vi "service new.vi"() -> ()   [LabVIEW 2009]
uses:
  <vilib>/printing/ReportDocExtensions.llb/Append Front Panel Image to Report (path).vi
  <vilib>/Utility/NIReport.llb/NI_report.lvclass
  <vilib>/Utility/NIReport.llb/NI_ReportGenerationCore.lvlib
panel:
  out "ALL":dbl[](graph)
  out "Left 2":dbl[](graph)
  out "Right":dbl[](graph)
  out "Serve 4":dbl[](graph)
  out "Serve 5":dbl[](graph)
  out "Serve 1":dbl[](graph)
  out "Serve 6":dbl[](graph)
  out "Serve 7":dbl[](graph)
  out "Serve 2":dbl[](graph)
  out "Serve 8":dbl[](graph)
  out "Serve 9":dbl[](graph)
  out "Serve 3":dbl[](graph)
  in  "S1":bool
  in  "TL":bool
  in  "BR":bool
  in  "BL":bool
  in  "BM":bool
  in  "CR":bool
  in  "CM":bool
  in  "CL":bool
  in  "TR":bool
  in  "TM":bool
  in  "1":bool
  in  "2":bool
  in  "3":bool
  in  "S 2":bool
  in  "Code":bool
  in  "stop":bool
  in  "save file to":path=path "C:/Users/Sports Tech/Desktop/kokum/Service VI/SAVED FILES/results.doc"
  in  "String":string
  in  "reset":bool
  in  "Boolean":bool
  in  "SHOW 2 to 2":bool
  in  "SHOW 2 to 1":bool
  in  "SHOW 1 to 2":bool
  in  "SHOW 1 to 1":bool
  in  "Serving 2 to 2":bool
  in  "Serving 2 to 1":bool
  in  "Serving 1 to 2":bool
  in  "Serving 1 to 1":bool
  out "service from right2 to 2":dbl[][](array[numeric])
  out "service from right2 to 1":dbl[][](array[numeric])
  out "service from right1 to 2":dbl[][](array[numeric])
  out "serving from left2 to 2":dbl[][](array[numeric])
  out "serving from left2 to 1":dbl[][](array[numeric])
  out "serving from left1 to 2":dbl[][](array[numeric])
  in  "TEAM 2 Player 2":string
  in  "TEAM 2 Player 1":string
  in  "TEAM 1 Player 2":string
  in  "TEAM 1 Player 1":string
  out "serve3":dbl[][](array[numeric])
  out "serve2":dbl[][](array[numeric])
  out "serve1":dbl[][](array[numeric])
  out "serv1 from right":dbl[][](array[numeric])
  out "serv2 from right":dbl[][](array[numeric])
  out "serv3 from right":dbl[][](array[numeric])
  out "serv3 from left":dbl[][](array[numeric])
  out "serv2 from left":dbl[][](array[numeric])
  out "serv1 from left":dbl[][](array[numeric])
  out "all serves":dbl[][](array[numeric])
  out "service from right1 to 1":dbl[][](array[numeric])
  out "serving from left1 to 1":dbl[][](array[numeric])
  # "SWITCH"
  # "Player position"
  # "Serving"
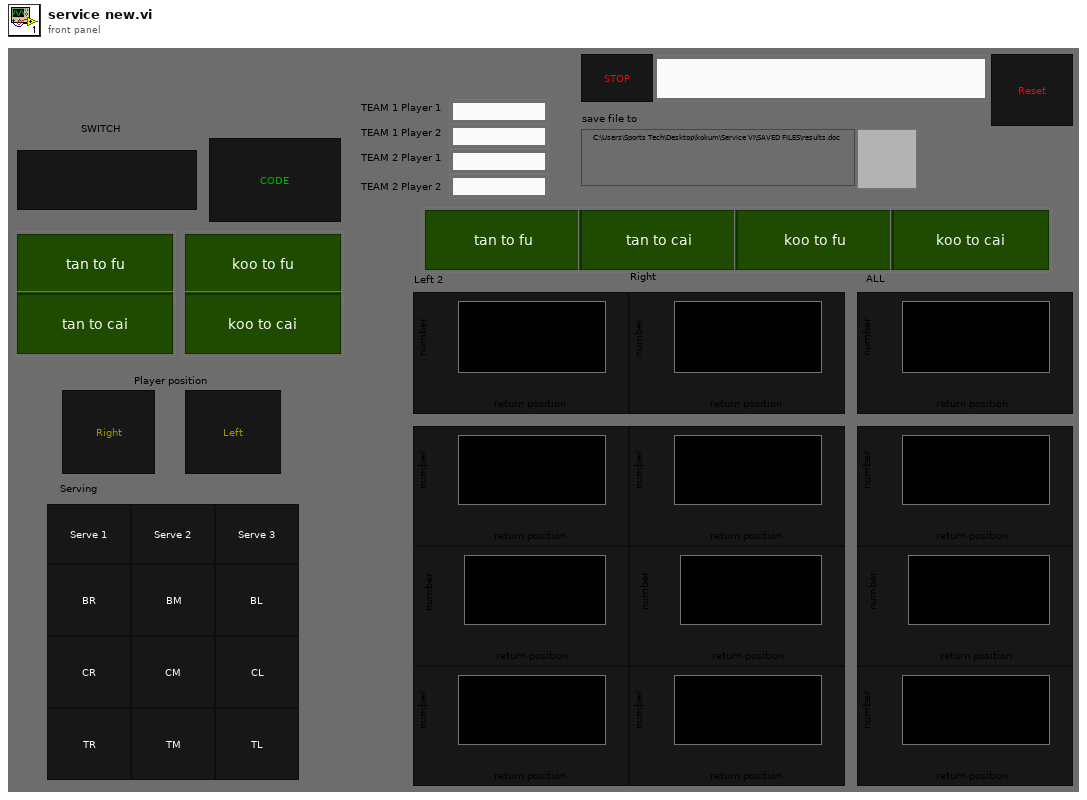
[diagram p1: front panel]
types:
  T1 = typedef "LVPositionTypeDef.ctl" = cluster{"Left":i32, "Top":i32}
  T2 = cluster{"Position":T1, "Position":T1, "Position":T1, "Position":T1, "Position":T1, "Position":T1, "Position":T1, "Position":T1, "Position":T1}
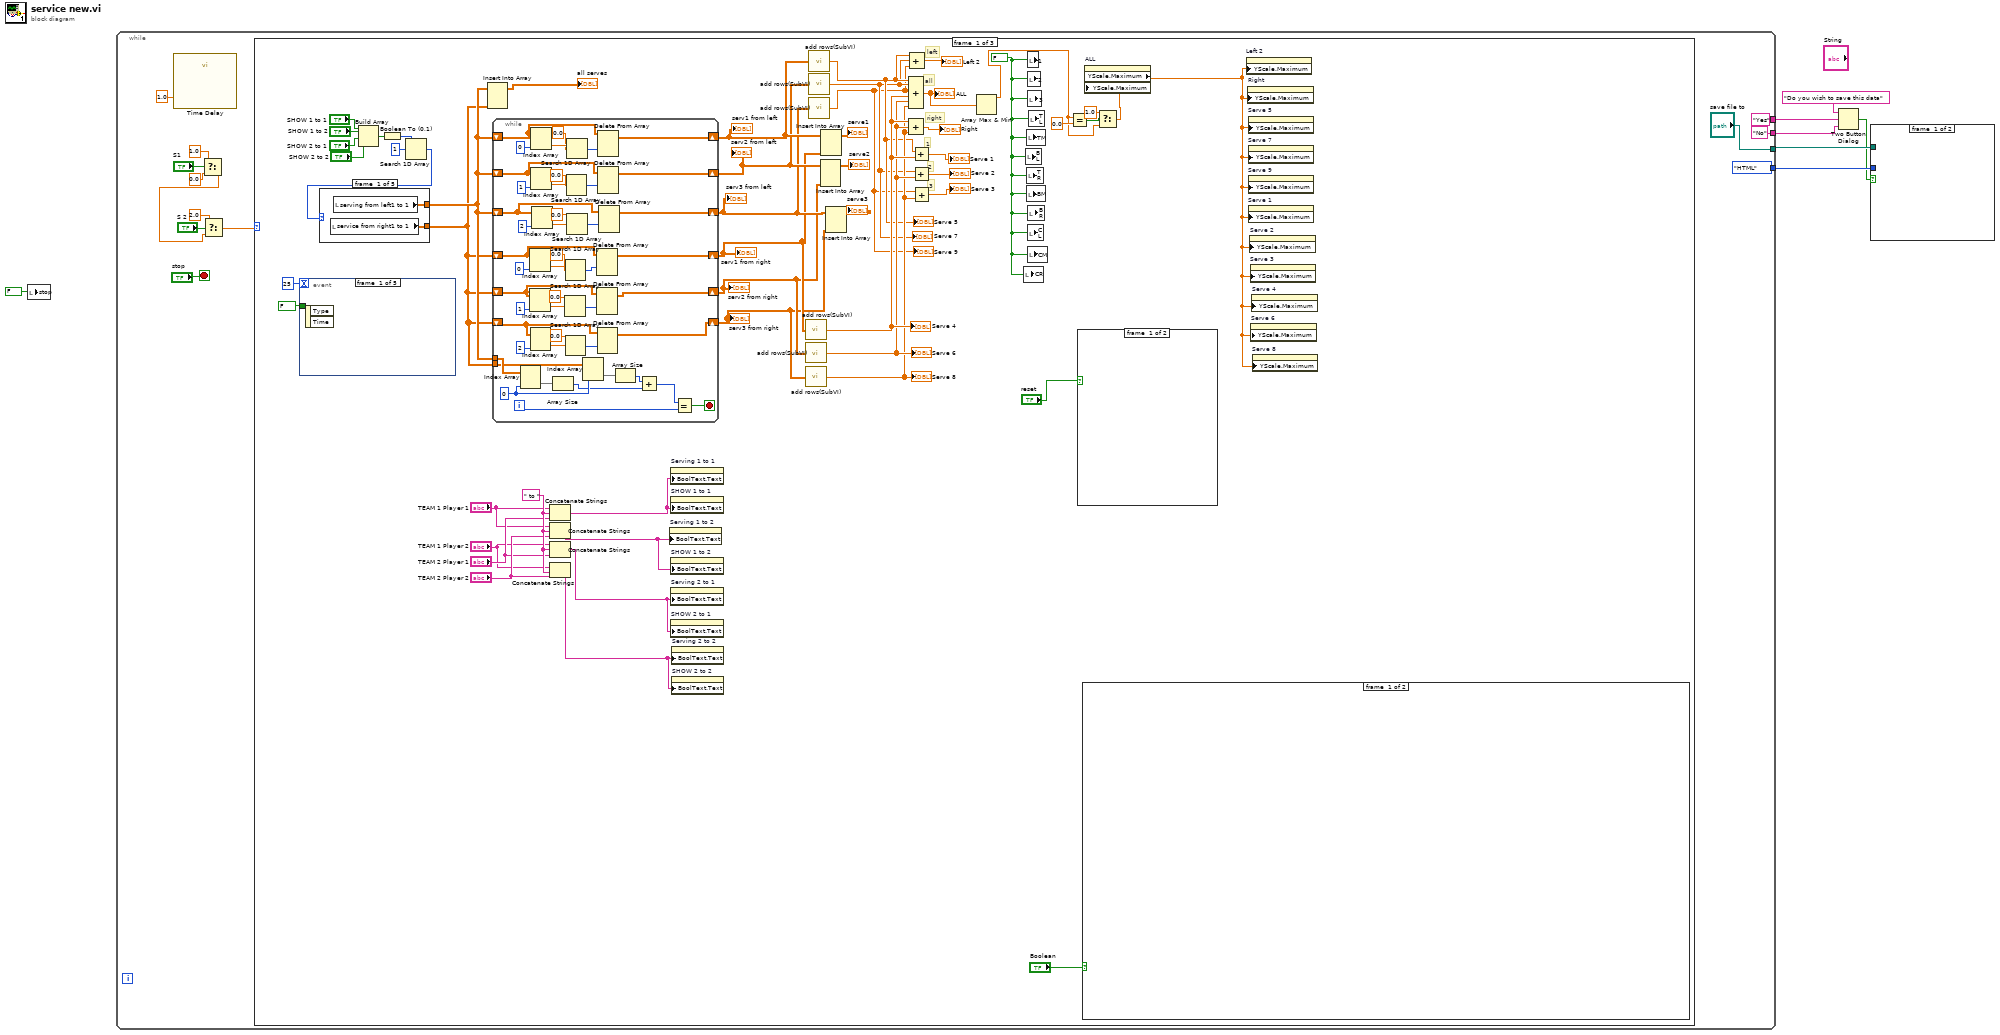
[diagram p0: block diagram]
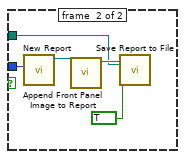
[diagram p2: hidden frame]
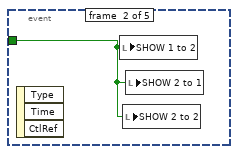
[diagram p3: hidden frame]
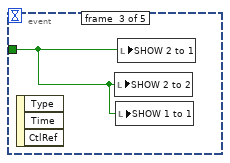
[diagram p4: hidden frame]
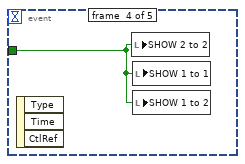
[diagram p5: hidden frame]
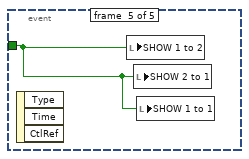
[diagram p6: hidden frame]
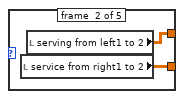
[diagram p7: hidden frame]
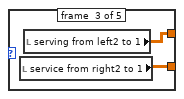
[diagram p8: hidden frame]
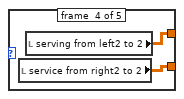
[diagram p9: hidden frame]
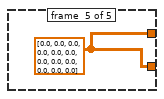
[diagram p10: hidden frame]
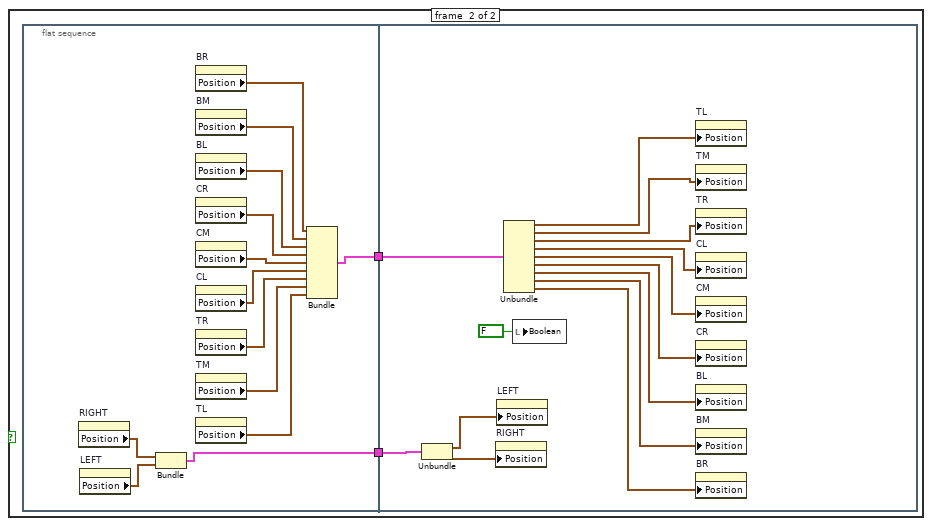
[diagram p11: hidden frame]
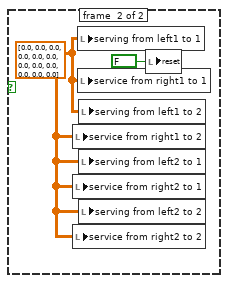
[diagram p12: hidden frame]
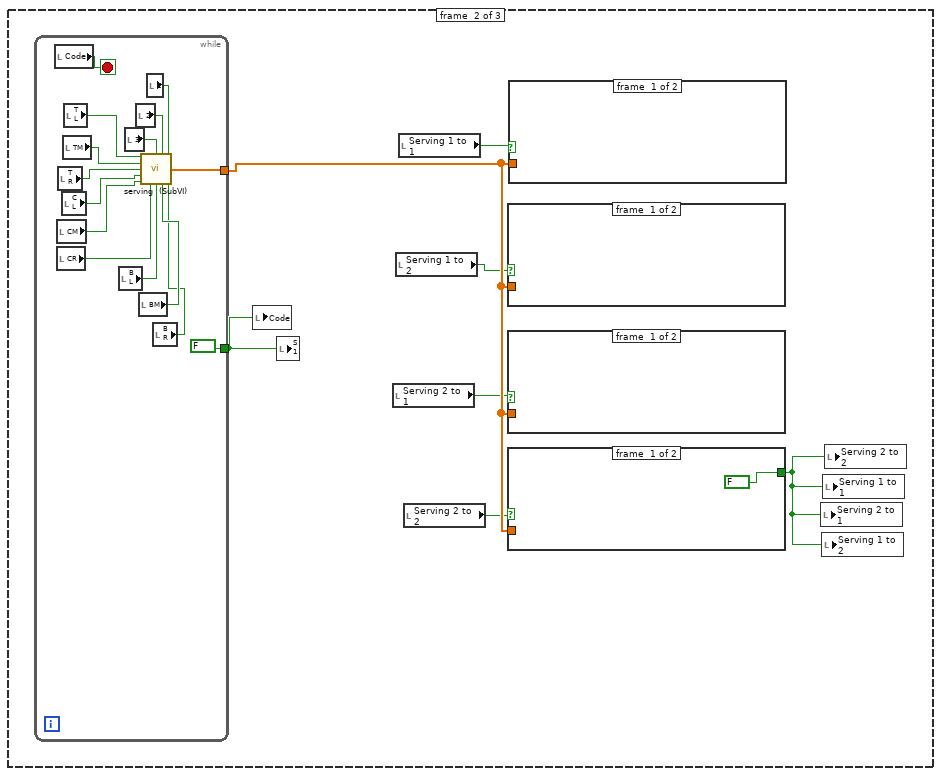
[diagram p13: hidden frame]
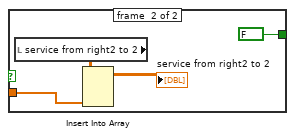
[diagram p14: hidden frame]
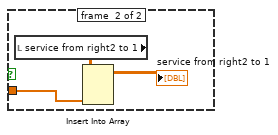
[diagram p15: hidden frame]
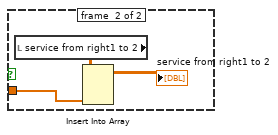
[diagram p16: hidden frame]
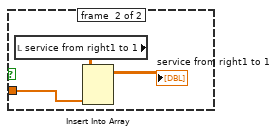
[diagram p17: hidden frame]
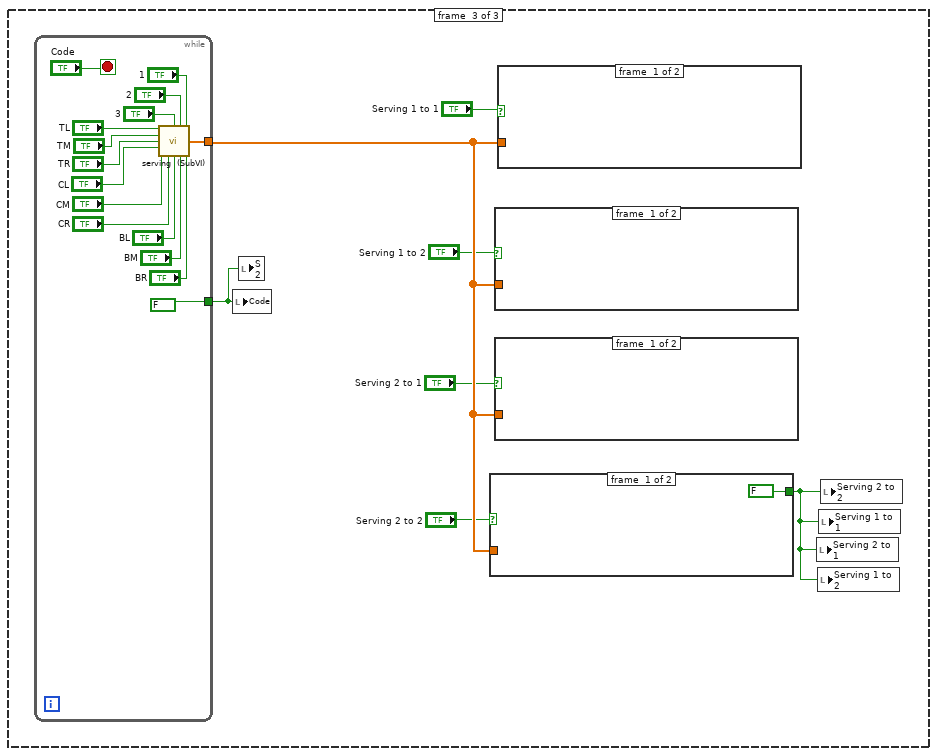
[diagram p18: hidden frame]
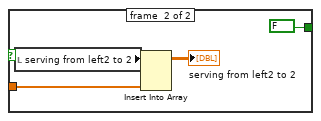
[diagram p19: hidden frame]
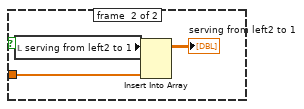
[diagram p20: hidden frame]
diagram:
  n1 = local write "stop"(FALSE ("stop")) -> ()
  n2 = while {
    tunnel: [enum16{"Standard Report", "HTML"}."HTML" ("report type")] -> w7
    tunnel: ["save file to"] -> w6
    tunnel: ["Yes" ("T button name (\"OK\")")] -> w3
    tunnel: ["No" ("F button name (\"Cancel\")")] -> w2
    stop <- "stop" stop-if-true
    n3 = call "Time Delay"("Delay Time (s)"=1.0) -> ()  [unwired: 10 in, 1 out]
    n4 = Select(t=1.0, s="S1", f=0.0) -> (s? t:f=w15:dbl)
    n5 = Select(t=2.0, s="S 2", f=w15) -> (s? t:f=w13:dbl)
    n6 = case shown="0, Default" w13 {
      frame #0 {
        w37 = " to " ("string")
        w51 = FALSE ("1")
        # "3"
        # "2"
        # "1"
        # "all"
        # "right"
        # "left"
        n7 = event shown="[4] \"SHOW 2 to 2\": Value Change" {
          selector: _ -> [_ _ _ _ _]
          dyn-events: _ -> [_ _ _ _ _]
          timeout: 25 -> [_ _ _ _ _]
          tunnel: FALSE ("SHOW 1 to 2") -> [_ w73 w74 w75 w76]
          event #0 {
            n8 = event-data() -> ()  [unwired: 1 in, 2 out]
          }
          event #1 {
            n9 = event-data() -> ()  [unwired: 1 in, 3 out]
            n10 = local write "SHOW 1 to 2"(w73) -> ()
            n11 = local write "SHOW 2 to 2"(w73) -> ()
            n12 = local write "SHOW 2 to 1"(w73) -> ()
          }
          event #2 {
            n13 = event-data() -> ()  [unwired: 1 in, 3 out]
            n14 = local write "SHOW 2 to 2"(w74) -> ()
            n15 = local write "SHOW 1 to 1"(w74) -> ()
            n16 = local write "SHOW 2 to 1"(w74) -> ()
          }
          event #3 {
            n17 = event-data() -> ()  [unwired: 1 in, 3 out]
            n18 = local write "SHOW 2 to 2"(w75) -> ()
            n19 = local write "SHOW 1 to 1"(w75) -> ()
            n20 = local write "SHOW 1 to 2"(w75) -> ()
          }
          event #4 {
            n21 = event-data() -> ()  [unwired: 1 in, 3 out]
            n22 = local write "SHOW 1 to 2"(w76) -> ()
            n23 = local write "SHOW 2 to 1"(w76) -> ()
            n24 = local write "SHOW 1 to 1"(w76) -> ()
          }
        }
        n25 = Build Array("SHOW 1 to 1", "SHOW 1 to 2", "SHOW 2 to 1", "SHOW 2 to 2") -> (w28:bool[])
        n26 = Boolean To (0,1)(Boolean=w28) -> (0, 1=w27:i16[])
        n27 = Search 1D Array(1D array=w27, element=i16 1) -> (index of element=w25:i32)  [unwired: 1 in]
        n28 = case shown="3" w25 {
          tunnel: [w78 w80 w82 w84 w85] -> w24
          tunnel: [w77 w79 w81 w83 w85] -> w23
          frame #0 {
            n29 = local read "service from right1 to 1"() -> (w77:dbl[][])
            n30 = local read "serving from left1 to 1"() -> (w78:dbl[][])
          }
          frame #1 {
            n31 = local read "service from right1 to 2"() -> (w79:dbl[][])
            n32 = local read "serving from left1 to 2"() -> (w80:dbl[][])
          }
          frame #2 {
            n33 = local read "service from right2 to 1"() -> (w81:dbl[][])
            n34 = local read "serving from left2 to 1"() -> (w82:dbl[][])
          }
          frame #3 {
            n35 = local read "service from right2 to 2"() -> (w83:dbl[][])
            n36 = local read "serving from left2 to 2"() -> (w84:dbl[][])
          }
          frame #4 {
            w85 = dbl[][] [[0.0, 0.0, 0.0, 0.0, 0.0, 0.0, 0.0, 0.0, 0.0, 0.0, 0.0, 0.0]] ("serving from left")
          }
        }
        n37 = Insert Into Array(array=w24, new element=w23) -> (→"all serves":dbl[][])  [unwired: 2 in]
        n38 = while {
          shift-right: [w158] -> w68
          shift-left: w24 -> [w160]
          shift-right: [w151] -> w67
          shift-left: w24 -> [w152]
          shift-right: [w146] -> w66
          shift-left: w24 -> [w147]
          shift-right: [w126] -> w65
          shift-left: w23 -> [w129]
          shift-right: [w125] -> w64
          shift-left: w23 -> [w128]
          shift-right: [w124] -> w63
          shift-left: w23 -> [w127]
          tunnel: w24 -> [w123]
          tunnel: w23 -> [w121]
          i -> [w144]
          stop <- w143 stop-if-true
          w122 = 0 ("disabled index (col)")
          n39 = Index Array(array=w123, index (col)=w122) -> (element=w120:dbl[])  [unwired: 1 in]
          n40 = Index Array(array=w129, index (col)=0 ("disabled index (col)")) -> (element=w130:dbl[])  [unwired: 1 in]
          n41 = Index Array(array=w128, index (col)=1 ("disabled index (col)")) -> (element=w135:dbl[])  [unwired: 1 in]
          n42 = Index Array(array=w127, index (col)=2 ("disabled index (col)")) -> (element=w141:dbl[])  [unwired: 1 in]
          n43 = Index Array(array=w160, index (col)=0 ("disabled index (col)")) -> (element=w162:dbl[])  [unwired: 1 in]
          n44 = Index Array(array=w152, index (col)=1 ("disabled index (col)")) -> (element=w155:dbl[])  [unwired: 1 in]
          n45 = Index Array(array=w147, index (col)=2 ("disabled index (col)")) -> (element=w145:dbl[])  [unwired: 1 in]
          n46 = Array Size(array=w120) -> (size(s)=w118:i32)
          n47 = Search 1D Array(1D array=w135, element=0.0) -> (index of element=w133:i32)  [unwired: 1 in]
          n48 = Search 1D Array(1D array=w130, element=0.0) -> (index of element=w132:i32)  [unwired: 1 in]
          n49 = Search 1D Array(1D array=w141, element=0.0) -> (index of element=w139:i32)  [unwired: 1 in]
          n50 = Search 1D Array(1D array=w155, element=0.0) -> (index of element=w157:i32)  [unwired: 1 in]
          n51 = Search 1D Array(1D array=w162, element=0.0) -> (index of element=w159:i32)  [unwired: 1 in]
          n52 = Search 1D Array(1D array=w145, element=0.0) -> (index of element=w149:i32)  [unwired: 1 in]
          n53 = Index Array(array=w121, index (col)=w122) -> (element=w142:dbl[])  [unwired: 1 in]
          n54 = Delete From Array(array=w129, index (row)=w132) -> (array with subset deleted=w126:dbl[][])  [unwired: 2 in, 1 out]
          n55 = Delete From Array(array=w128, index (row)=w133) -> (array with subset deleted=w125:dbl[][])  [unwired: 2 in, 1 out]
          n56 = Delete From Array(array=w127, index (row)=w139) -> (array with subset deleted=w124:dbl[][])  [unwired: 2 in, 1 out]
          n57 = Delete From Array(array=w160, index (row)=w159) -> (array with subset deleted=w158:dbl[][])  [unwired: 2 in, 1 out]
          n58 = Delete From Array(array=w152, index (row)=w157) -> (array with subset deleted=w151:dbl[][])  [unwired: 2 in, 1 out]
          n59 = Delete From Array(array=w147, index (row)=w149) -> (array with subset deleted=w146:dbl[][])  [unwired: 2 in, 1 out]
          n60 = Array Size(array=w142) -> (size(s)=w119:i32)
          n61 = Add(x=w119, y=w118) -> (x+y=w117:i32)
          n62 = Equal?(x=w117, y=w144) -> (x = y?=w143:bool)
        }
        "serv1 from left" <- w68
        "serv2 from left" <- w67
        "serv3 from left" <- w66
        "serv1 from right" <- w65
        "serv2 from right" <- w64
        "serv3 from right" <- w63
        n63 = Concatenate Strings("TEAM 1 Player 1", w37, "TEAM 2 Player 1") -> (w38:string)
        n64 = Concatenate Strings("TEAM 1 Player 1", w37, "TEAM 2 Player 2") -> (w39:string)
        n65 = Concatenate Strings("TEAM 1 Player 2", w37, "TEAM 2 Player 1") -> (w40:string)
        n66 = Concatenate Strings("TEAM 1 Player 2", w37, "TEAM 2 Player 2") -> (w41:string)
        n67 = property on="Serving 1 to 2" class="Bool (strict)"("BoolText.Text"=w39) -> ()  [unwired: 2 in, 2 out]
        n68 = property on="Serving 1 to 1" class="Bool (strict)"("BoolText.Text"=w38) -> ()  [unwired: 2 in, 2 out]
        n69 = property on="SHOW 1 to 1" class="Bool (strict)"("BoolText.Text"=w38) -> ()  [unwired: 2 in, 2 out]
        n70 = property on="SHOW 1 to 2" class="Bool (strict)"("BoolText.Text"=w39) -> ()  [unwired: 2 in, 2 out]
        n71 = property on="Serving 2 to 1" class="Bool (strict)"("BoolText.Text"=w40) -> ()  [unwired: 2 in, 2 out]
        n72 = property on="SHOW 2 to 1" class="Bool (strict)"("BoolText.Text"=w40) -> ()  [unwired: 2 in, 2 out]
        n73 = property on="Serving 2 to 2" class="Bool (strict)"("BoolText.Text"=w41) -> ()  [unwired: 2 in, 2 out]
        n74 = property on="SHOW 2 to 2" class="Bool (strict)"("BoolText.Text"=w41) -> ()  [unwired: 2 in, 2 out]
        n75 = call "add rows(SubVI).vi"("array in"=w65) -> ("array out"=w62:dbl[])
        "Serve 4" <- w62
        n76 = call "add rows(SubVI).vi"("array in"=w64) -> ("array out"=w61:dbl[])
        "Serve 6" <- w61
        n77 = call "add rows(SubVI).vi"("array in"=w63) -> ("array out"=w60:dbl[])
        "Serve 8" <- w60
        n78 = call "add rows(SubVI).vi"("array in"=w68) -> ("array out"=w59:dbl[])
        "Serve 5" <- w59
        n79 = call "add rows(SubVI).vi"("array in"=w67) -> ("array out"=w58:dbl[])
        "Serve 7" <- w58
        n80 = call "add rows(SubVI).vi"("array in"=w66) -> ("array out"=w57:dbl[])
        "Serve 9" <- w57
        n81 = Insert Into Array(array=w67, new element=w64) -> (→"serve2":dbl[][])  [unwired: 2 in]
        n82 = Insert Into Array(array=w68, new element=w65) -> (→"serve1":dbl[][])  [unwired: 2 in]
        n83 = Insert Into Array(array=w66, new element=w63) -> (→"serve3":dbl[][])  [unwired: 2 in]
        n84 = Compound Arithmetic op=ADD(w59, w58, w57, w62, w61, w60) -> (w49:dbl[])
        "ALL" <- w49
        n85 = Compound Arithmetic op=ADD(w62, w61, w60) -> (→"Right":dbl[])
        n86 = Compound Arithmetic op=ADD(w59, w58, w57) -> (→"Left 2":dbl[])
        n87 = Add(x=w59, y=w62) -> (x+y=→"Serve 1":dbl[])
        n88 = Add(x=w58, y=w61) -> (x+y=→"Serve 2":dbl[])
        n89 = Add(x=w57, y=w60) -> (x+y=→"Serve 3":dbl[])
        n90 = Array Max & Min(array=w49) -> (max value=w45:dbl)  [unwired: 3 out]
        n91 = local write "CR"(w51) -> ()
        n92 = local write "BL"(w51) -> ()
        n93 = local write "TM"(w51) -> ()
        n94 = local write "TR"(w51) -> ()
        n95 = local write "BM"(w51) -> ()
        n96 = local write "1"(w51) -> ()
        n97 = local write "2"(w51) -> ()
        n98 = local write "CL"(w51) -> ()
        n99 = local write "CM"(w51) -> ()
        n100 = local write "3"(w51) -> ()
        n101 = local write "BR"(w51) -> ()
        n102 = local write "TL"(w51) -> ()
        n103 = Equal?(x=w45, y=0.0) -> (x = y?=w47:bool)
        n104 = case shown="True" "reset" {
          frame #0 {
          }
          frame #1 {
            w115 = dbl[][] [[0.0, 0.0, 0.0, 0.0, 0.0, 0.0, 0.0, 0.0, 0.0, 0.0, 0.0, 0.0]] ("serving from left")
            n105 = local write "service from right1 to 2"(w115) -> ()
            n106 = local write "service from right2 to 1"(w115) -> ()
            n107 = local write "service from right2 to 2"(w115) -> ()
            n108 = local write "serving from left1 to 1"(w115) -> ()
            n109 = local write "service from right1 to 1"(w115) -> ()
            n110 = local write "serving from left1 to 2"(w115) -> ()
            n111 = local write "serving from left2 to 1"(w115) -> ()
            n112 = local write "serving from left2 to 2"(w115) -> ()
            n113 = local write "reset"(FALSE ("reset")) -> ()
          }
        }
        n114 = case shown="True" "Boolean" {
          frame #0 {
          }
          frame #1 {
            n115 = flat-sequence {
              tunnel: [w89] -> w87
              tunnel: [w88] -> w86
              tunnel: w87 -> [w114]
              tunnel: w86 -> [w104]
              frame #0 {
                n116 = property on="RIGHT" class="Bool (strict)"() -> ("Position"=w90:T1)  [unwired: 2 in, 2 out]
                n117 = property on="LEFT" class="Bool (strict)"() -> ("Position"=w91:T1)  [unwired: 2 in, 2 out]
                n118 = Bundle("Position"=w90, "Position"=w91) -> (w88:cluster{"Position":T1, "Position":T1})  [unwired: 1 in]
                n119 = property on="BR" class="Bool (strict)"() -> ("Position"=w100:T1)  [unwired: 2 in, 2 out]
                n120 = property on="BM" class="Bool (strict)"() -> ("Position"=w99:T1)  [unwired: 2 in, 2 out]
                n121 = property on="BL" class="Bool (strict)"() -> ("Position"=w98:T1)  [unwired: 2 in, 2 out]
                n122 = property on="CR" class="Bool (strict)"() -> ("Position"=w97:T1)  [unwired: 2 in, 2 out]
                n123 = property on="CM" class="Bool (strict)"() -> ("Position"=w96:T1)  [unwired: 2 in, 2 out]
                n124 = property on="CL" class="Bool (strict)"() -> ("Position"=w95:T1)  [unwired: 2 in, 2 out]
                n125 = property on="TR" class="Bool (strict)"() -> ("Position"=w94:T1)  [unwired: 2 in, 2 out]
                n126 = property on="TM" class="Bool (strict)"() -> ("Position"=w93:T1)  [unwired: 2 in, 2 out]
                n127 = property on="TL" class="Bool (strict)"() -> ("Position"=w92:T1)  [unwired: 2 in, 2 out]
                n128 = Bundle("Position"=w100, "Position"=w99, "Position"=w98, "Position"=w97, "Position"=w96, "Position"=w95, "Position"=w94, "Position"=w93, "Position"=w92) -> (w89:T2)  [unwired: 1 in]
              }
              frame #1 {
                n129 = Unbundle(w104) -> ("Position"=w103:T1, "Position"=w102:T1)
                n130 = property on="RIGHT" class="Bool (strict)"("Position"=w102) -> ()  [unwired: 2 in, 2 out]
                n131 = property on="LEFT" class="Bool (strict)"("Position"=w103) -> ()  [unwired: 2 in, 2 out]
                n132 = Unbundle(w114) -> ("Position"=w113:T1, "Position"=w112:T1, "Position"=w111:T1, "Position"=w110:T1, "Position"=w109:T1, "Position"=w108:T1, "Position"=w107:T1, "Position"=w106:T1, "Position"=w105:T1)
                n133 = local write "Boolean"(FALSE ("Boolean")) -> ()
                n134 = property on="TL" class="Bool (strict)"("Position"=w113) -> ()  [unwired: 2 in, 2 out]
                n135 = property on="TM" class="Bool (strict)"("Position"=w112) -> ()  [unwired: 2 in, 2 out]
                n136 = property on="TR" class="Bool (strict)"("Position"=w111) -> ()  [unwired: 2 in, 2 out]
                n137 = property on="CL" class="Bool (strict)"("Position"=w110) -> ()  [unwired: 2 in, 2 out]
                n138 = property on="CM" class="Bool (strict)"("Position"=w109) -> ()  [unwired: 2 in, 2 out]
                n139 = property on="CR" class="Bool (strict)"("Position"=w108) -> ()  [unwired: 2 in, 2 out]
                n140 = property on="BL" class="Bool (strict)"("Position"=w107) -> ()  [unwired: 2 in, 2 out]
                n141 = property on="BM" class="Bool (strict)"("Position"=w106) -> ()  [unwired: 2 in, 2 out]
                n142 = property on="BR" class="Bool (strict)"("Position"=w105) -> ()  [unwired: 2 in, 2 out]
              }
            }
          }
        }
        n143 = Select(t=1.0, s=w47, f=w45) -> (s? t:f=w44:dbl)
        n144 = property on="ALL" class="WFGraph (strict)"("YScale.Maximum"=w44) -> ("YScale.Maximum"=w50:dbl)  [unwired: 2 in, 2 out]
        n145 = property on="Left 2" class="WFGraph (strict)"("YScale.Maximum"=w50) -> ()  [unwired: 2 in, 2 out]
        n146 = property on="Right" class="WFGraph (strict)"("YScale.Maximum"=w50) -> ()  [unwired: 2 in, 2 out]
        n147 = property on="Serve 5" class="WFGraph (strict)"("YScale.Maximum"=w50) -> ()  [unwired: 2 in, 2 out]
        n148 = property on="Serve 7" class="WFGraph (strict)"("YScale.Maximum"=w50) -> ()  [unwired: 2 in, 2 out]
        n149 = property on="Serve 9" class="WFGraph (strict)"("YScale.Maximum"=w50) -> ()  [unwired: 2 in, 2 out]
        n150 = property on="Serve 1" class="WFGraph (strict)"("YScale.Maximum"=w50) -> ()  [unwired: 2 in, 2 out]
        n151 = property on="Serve 2" class="WFGraph (strict)"("YScale.Maximum"=w50) -> ()  [unwired: 2 in, 2 out]
        n152 = property on="Serve 3" class="WFGraph (strict)"("YScale.Maximum"=w50) -> ()  [unwired: 2 in, 2 out]
        n153 = property on="Serve 6" class="WFGraph (strict)"("YScale.Maximum"=w50) -> ()  [unwired: 2 in, 2 out]
        n154 = property on="Serve 4" class="WFGraph (strict)"("YScale.Maximum"=w50) -> ()  [unwired: 2 in, 2 out]
        n155 = property on="Serve 8" class="WFGraph (strict)"("YScale.Maximum"=w50) -> ()  [unwired: 2 in, 2 out]
      }
      frame #1 {
        n156 = while {
          tunnel: [w186] -> w168
          tunnel: [FALSE ("S1")] -> w169
          stop <- w198 stop-if-true
          n157 = local read "Code"() -> (w198:bool)
          n158 = local read "CM"() -> (w193:bool)
          n159 = local read "CR"() -> (w194:bool)
          n160 = local read "TR"() -> (w184:bool)
          n161 = local read "CL"() -> (w192:bool)
          n162 = local read "TM"() -> (w191:bool)
          n163 = local read "TL"() -> (w190:bool)
          n164 = local read "BL"() -> (w197:bool)
          n165 = local read "3"() -> (w189:bool)
          n166 = local read "2"() -> (w188:bool)
          n167 = local read "BM"() -> (w196:bool)
          n168 = local read "1"() -> (w187:bool)
          n169 = local read "BR"() -> (w195:bool)
          n170 = call "serving  (SubVI).vi"("1"=w187, "BR"=w195, "2"=w188, "BM"=w196, "3"=w189, "BL"=w197, "CR"=w194, "TL"=w190, "TM"=w191, "TR"=w184, "CL"=w192, "CM"=w193) -> ("appended array"=w186:dbl[])  [unwired: 3 in]
        }
        n171 = local write "Code"(w169) -> ()
        n172 = local write "S1"(w169) -> ()
        n173 = local read "Serving 2 to 1"() -> (w165:bool)
        n174 = local read "Serving 1 to 2"() -> (w166:bool)
        n175 = local read "Serving 1 to 1"() -> (w167:bool)
        n176 = local read "Serving 2 to 2"() -> (w164:bool)
        n177 = case shown="True" w166 {
          tunnel: w168 -> [_ w178]
          frame #0 {
          }
          frame #1 {
            n178 = local read "service from right1 to 2"() -> (w180:dbl[][])
            n179 = Insert Into Array(array=w180, new element=w178) -> (→"service from right1 to 2":dbl[][])  [unwired: 2 in]
          }
        }
        n180 = case shown="True" w165 {
          tunnel: w168 -> [_ w175]
          frame #0 {
          }
          frame #1 {
            n181 = local read "service from right2 to 1"() -> (w177:dbl[][])
            n182 = Insert Into Array(array=w177, new element=w175) -> (→"service from right2 to 1":dbl[][])  [unwired: 2 in]
          }
        }
        n183 = case shown="True" w164 {
          tunnel: w168 -> [_ w172]
          tunnel: [FALSE ("S1") FALSE ("S1")] -> w163
          frame #0 {
          }
          frame #1 {
            n184 = local read "service from right2 to 2"() -> (w174:dbl[][])
            n185 = Insert Into Array(array=w174, new element=w172) -> (→"service from right2 to 2":dbl[][])  [unwired: 2 in]
          }
        }
        n186 = case shown="True" w167 {
          tunnel: w168 -> [_ w181]
          frame #0 {
          }
          frame #1 {
            n187 = local read "service from right1 to 1"() -> (w183:dbl[][])
            n188 = Insert Into Array(array=w183, new element=w181) -> (→"service from right1 to 1":dbl[][])  [unwired: 2 in]
          }
        }
        n189 = local write "Serving 2 to 1"(w163) -> ()
        n190 = local write "Serving 1 to 2"(w163) -> ()
        n191 = local write "Serving 1 to 1"(w163) -> ()
        n192 = local write "Serving 2 to 2"(w163) -> ()
      }
      frame #2 {
        n193 = while {
          tunnel: [w221] -> w203
          tunnel: [FALSE ("S 2")] -> w205
          stop <- "Code" stop-if-true
          n194 = call "serving  (SubVI).vi"("1"="1", "BR"="BR", "2"="2", "BM"="BM", "3"="3", "BL"="BL", "CR"="CR", "TL"="TL", "TM"="TM", "TR"="TR", "CL"="CL", "CM"="CM") -> ("appended array"=w221:dbl[])  [unwired: 3 in]
        }
        n195 = local write "Code"(w205) -> ()
        n196 = local write "S 2"(w205) -> ()
        n197 = case shown="True" "Serving 2 to 2" {
          tunnel: w203 -> [_ w208]
          tunnel: [FALSE ("Serving 2 to 2") FALSE ("Serving 2 to 2")] -> w199
          frame #0 {
          }
          frame #1 {
            n198 = local read "serving from left2 to 2"() -> (w210:dbl[][])
            n199 = Insert Into Array(array=w210, new element=w208) -> (→"serving from left2 to 2":dbl[][])  [unwired: 2 in]
          }
        }
        n200 = case shown="True" "Serving 1 to 2" {
          tunnel: w203 -> [_ w214]
          frame #0 {
          }
          frame #1 {
            n201 = local read "serving from left1 to 2"() -> (w216:dbl[][])
            n202 = Insert Into Array(array=w216, new element=w214) -> (→"serving from left1 to 2":dbl[][])  [unwired: 2 in]
          }
        }
        n203 = case shown="True" "Serving 2 to 1" {
          tunnel: w203 -> [_ w211]
          frame #0 {
          }
          frame #1 {
            n204 = local read "serving from left2 to 1"() -> (w213:dbl[][])
            n205 = Insert Into Array(array=w213, new element=w211) -> (→"serving from left2 to 1":dbl[][])  [unwired: 2 in]
          }
        }
        n206 = case shown="True" "Serving 1 to 1" {
          tunnel: w203 -> [_ w217]
          frame #0 {
          }
          frame #1 {
            n207 = local read "serving from left1 to 1"() -> (w219:dbl[][])
            n208 = Insert Into Array(array=w219, new element=w217) -> (→"serving from left1 to 1":dbl[][])  [unwired: 2 in]
          }
        }
        n209 = local write "Serving 2 to 1"(w199) -> ()
        n210 = local write "Serving 1 to 2"(w199) -> ()
        n211 = local write "Serving 1 to 1"(w199) -> ()
        n212 = local write "Serving 2 to 2"(w199) -> ()
      }
    }
  }
  n213 = Two Button Dialog(message="Do you wish to save this data", 1:w2, 2:w3) -> (T button?=w4:bool)
  n214 = case shown="True" w4 {
    tunnel: w7 -> [_ w239]
    tunnel: w6 -> [_ w236]
    frame #0 {
    }
    frame #1 {
      n215 = call <vilib>:"New Report.vi"("report type"=w239) -> ("report out"=w238:refnum<class "NI_report.lvclass">)  [unwired: 13 in, 1 out]
      n216 = call-poly <vilib>:"Append Front Panel Image to Report.vi"("report in"=w238) -> ("report out"=w237:refnum<class "NI_report.lvclass">)  [unwired: 10 in, 4 out]
      n217 = call-dynamic "Save Report to File.vi"("report in"=w237, "report file path"=w236, "prompt to replace? (F)"=TRUE ("Prompt to Replace? (F)")) -> ()  [unwired: 11 in, 2 out]
    }
  }
